vi "New VI From Template.vi"(6 "Mouse Position":T1, 7 "User VI Ref":refnum<vi>, 8 "Is Multi-select?":bool, 9 "Remaining Items":refnum<vi>[](array[refnum]), 10 "Affected Items":cluster{"Any Refnums":refnum<vi>[]}, 11 "Menu Refnum":refnum<k9>) -> (3 "Menu Items To Add":T2[](array[typedef]))   [LabVIEW 2021]
doc: "Adds the Menu Item \"New VI...\" when a single free label (comment) was right-clicked on the block diagram or on the front panel.\n\nDoes nothing if two or more free labels were selected."
uses:
  <resource>/plugins/PopupMenus/support/Shortcut Menu Item Definition.ctl
  <resource>/plugins/PopupMenus/support/Transaction Control.ctl
  <resource>/plugins/PopupMenus/support/Position In Menu.ctl
  <resource>/plugins/PopupMenus/support/Relative Position.ctl
  <resource>/plugins/PopupMenus/support/Checkmark Status.ctl
  <resource>/plugins/PopupMenus/support/Enabled Menu Item Status.ctl
  <vilib>/Utility/miscctls.llb/LVPositionTypeDef.ctl
panel:
  # "Rules a popup plug-in must follow:\n* This VI's file name must match the file name of the LLB -- only the file extensions should be different.\n* This VI must have debugging disabled or it will be ignored as a plug-in.\n* For all menu items, \"tag suffix + file name of this VI\" must be less than 240 characters.\n* You can disconnect the \"Affected Items\" from the typedef to make the plug-in load faster. The typedef is only there to assist you in keeping this VI and the execution VI using to the same type.\n* All controls on this panel except \"Affected Items\" are locked to prevent accidental edits. Do not change the types or the names of controls other than the elements inside the \"Affected Items\" cluster.\n* See Context Help for more information on the individual controls."
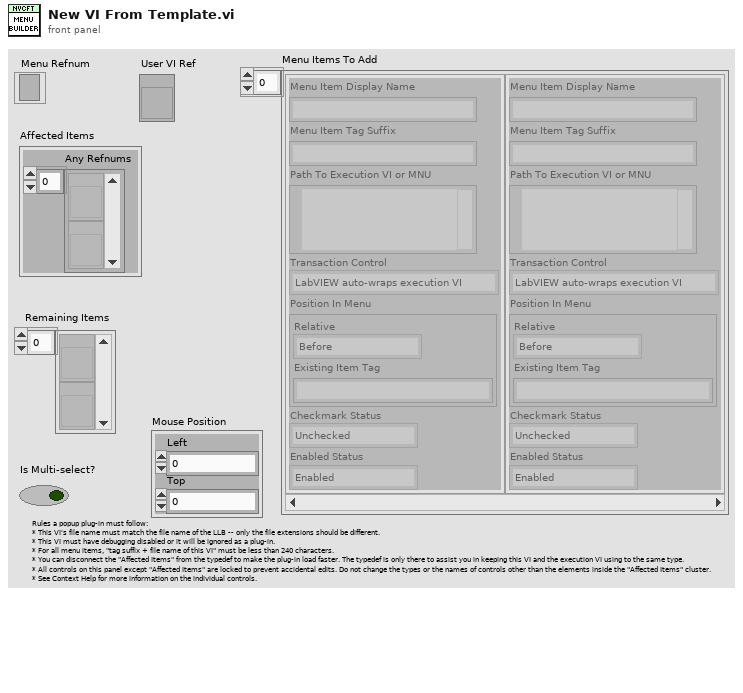
[diagram p1: front panel]
types:
  T1 = typedef "LVPositionTypeDef.ctl" = cluster{"Left":i32, "Top":i32}
  T2 = typedef "Shortcut Menu Item Definition.ctl" = cluster{"Menu Item Display Name":string, "Menu Item Tag Suffix":string, "Path To Execution VI or MNU":path, "Transaction Control":T3, "Position In Menu":T4, "Checkmark Status":T6, "Enabled Status":T7}
  T3 = typedef "Transaction Control.ctl" = enum8{"LabVIEW auto-wraps execution VI", "Execution VI will define if needed"}
  T4 = typedef "Position In Menu.ctl" = cluster{"Relative":T5, "Existing Item Tag":string}
  T5 = typedef "Relative Position.ctl" = enum8{"Before", "Instead of", "After", "Into Submenu"}
  T6 = typedef "Checkmark Status.ctl" = enum8{"Unchecked", "Checked"}
  T7 = typedef "Enabled Menu Item Status.ctl" = enum8{"Enabled", "Disabled"}
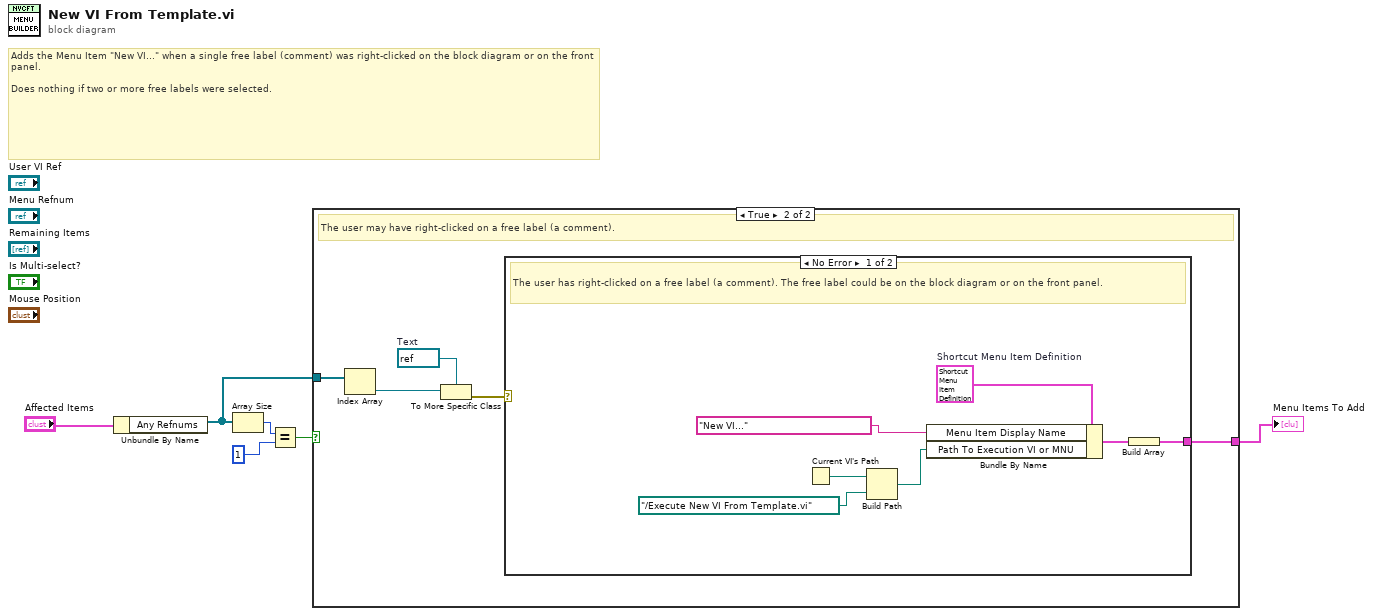
[diagram p0: block diagram]
diagram:
  # "Adds the Menu Item \"New VI...\" when a single free label (comment) was right-clicked on the block diagram or on the front panel.\n\nDoes nothing if two or more free labels were selected."
  n1 = Unbundle By Name("Affected Items") -> ("Any Refnums"=w2:refnum<vi>[])
  n2 = Array Size(array=w2) -> (size(s)=w5:i32)
  n3 = Equal?(x=w5, y=1) -> (x = y?=w3:bool)
  n4 = case shown="True" w3 {
    tunnel: w2 -> [_ w11]
    tunnel: [_ w7] -> w1
    frame False {
      # "The user has right-clicked on something other than a single free label (a comment)."
    }
    frame True {
      w10 = refnum<vi> refnum  # Text
      # "The user may have right-clicked on a free label (a comment)."
      n5 = Index Array(array=w11) -> (element=w9:refnum<vi>)  [unwired: 1 in]
      n6 = To More Specific Class(target class=w10, reference=w9) -> (error out=w8:errorcluster)  [unwired: 1 in, 1 out]
      n7 = case shown="No Error" w8 {
        tunnel: [w12 _] -> w7
        frame No Error {
          w14 = T2 {"Menu Item Display Name"="", "Menu Item Tag Suffix"="", "Path To Execution VI or MNU"=path "", "Transaction Control"=enum."Execution VI will define if needed", "Position In Menu"={"Relative"=enum."Before", "Existing Item Tag"=""}, "Checkmark Status"=enum."Unchecked", "Enabled Status"=enum."Enabled"}  # Shortcut Menu Item Definition
          # "The user has right-clicked on a free label (a comment). The free label could be on the block diagram or on the front panel."
          n8 = Current VI's Path() -> (path=w18:path)
          n9 = Build Path(base path=w18, name or relative path=path "../Execute New VI From Template.vi" ("execute path")) -> (appended path=w16:path)
          n10 = Bundle By Name(cluster=w14, "Menu Item Display Name"="New VI...", "Path To Execution VI or MNU"=w16) -> (w17:T2)
          n11 = Build Array(w17) -> (w12:T2[])
        }
        frame Error {
          # "The user has right-clicked on something other than a single free label (a comment)."
        }
      }
    }
  }
  "Menu Items To Add" <- w1
